vi "Rotate Point.vi"(9 "Rotation Angle (degree)":dbl, 10 "Center":cluster{"X":i32, "Y":i32}, 11 "Point in":cluster{"X":i32, "Y":i32}) -> (3 "Point out":cluster{"X":i32, "Y":i32})   [LabVIEW 2020, in "Map Model.lvlib" / "Map Model.lvclass"]
uses:
  Map Model.lvclass
panel:
  # "NOTICE -- YOU MUST LEAVE THIS NOTICE IN PLACE.\n\nCopyright (c) 2017, LIANG LIU Shawn.Liu.cn@gmail.com\nAll rights reserved.\n\nRedistribution and use in source and binary forms, with or without modification, are permitted provided that the following conditions are met:\n-Redistributions of source code must retain the above copyright notice, this list of conditions and the following disclaimer.\n-Redistributions in binary form must reproduce the above copyright notice, this list of conditions and the following disclaimer in the documentation and/or other materials provided with the distribution.\n-Neither the name of the eLp nor the names of its contributors may be used to endorse or promote products derived from this software without specific prior written permission.\n\nTHIS SOFTWARE IS PROVIDED BY THE COPYRIGHT HOLDERS AND CONTRIBUTORS \"AS IS\" AND ANY EXPRESS OR IMPLIED WARRANTIES, INCLUDING, BUT NOT LIMITED TO, THE IMPLIED WARRANTIES OF MERCHANTABILITY AND FITNESS FOR A PARTICULAR PURPOSE ARE DISCLAIMED. IN NO EVENT SHALL THE COPYRIGHT HOLDER OR CONTRIBUTORS BE LIABLE FOR ANY DIRECT, INDIRECT, INCIDENTAL, SPECIAL, EXEMPLARY, OR CONSEQUENTIAL DAMAGES (INCLUDING, BUT NOT LIMITED TO, PROCUREMENT OF SUBSTITUTE GOODS OR SERVICES; LOSS OF USE, DATA, OR PROFITS; OR BUSINESS INTERRUPTION) HOWEVER CAUSED AND ON ANY THEORY OF LIABILITY, WHETHER IN CONTRACT, STRICT LIABILITY, OR TORT (INCLUDING NEGLIGENCE OR OTHERWISE) ARISING IN ANY WAY OUT OF THE USE OF THIS SOFTWARE, EVEN IF ADVISED OF THE POSSIBILITY OF SUCH DAMAGE."
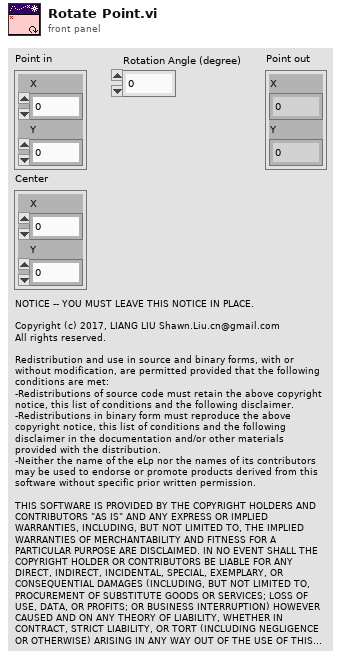
[diagram p1: front panel]
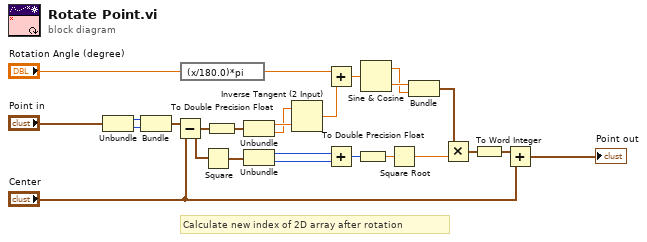
[diagram p0: block diagram]
diagram:
  # "Calculate new index of 2D array after rotation"
  n1 = Unbundle("Point in") -> ("X"=w6:i32, "Y"=w5:i32)
  n2 = Bundle("X"=w6, "Y"=w5) -> (w25:cluster{"X":i32, "Y":i32})  [unwired: 1 in]
  n3 = Subtract(x=w25, y="Center") -> (x-y=w10:cluster{"X":i32, "Y":i32})
  n4 = expression code="(x/180.0)*pi" ("degrees to radians")("Rotation Angle (degree)") -> (w2:dbl)
  n5 = Square(x=w10) -> (x^2=w24:cluster{"X":i32, "Y":i32})
  n6 = To Double Precision Float(number=w10) -> (double precision float=w9:cluster{"X":dbl, "Y":dbl})
  n7 = Unbundle(w9) -> ("X"=w20:dbl, "Y"=w19:dbl)
  n8 = Unbundle(w24) -> ("X"=w23:i32, "Y"=w22:i32)
  n9 = Inverse Tangent (2 Input)(1:w20, 2:w19) -> (0:w18:dbl)
  n10 = Add(x=w2, y=w18) -> (x+y=w17:dbl)
  n11 = Add(x=w23, y=w22) -> (x+y=w21:i32)
  n12 = To Double Precision Float(number=w21) -> (double precision float=w8:dbl)
  n13 = Sine & Cosine(0:w17) -> (1:w15:dbl, 2:w16:dbl)
  n14 = Square Root(x=w8) -> (sqrt(x)=w13:dbl)
  n15 = Bundle(w16, w15) -> (w14:cluster{dbl, dbl})  [unwired: 1 in]
  n16 = Multiply(x=w14, y=w13) -> (x*y=w12:cluster{dbl, dbl})
  n17 = To Word Integer(number=w12) -> (16bit integer=w11:cluster{i16, i16})
  n18 = Add(x=w11, y="Center") -> (x+y=→"Point out":cluster{i32, i32})
